vi "Configure Multitone.vi"(0 "VISA resource name":refnum<visa-resource-name>, 1 "Multitone Signal Length (0: ml512)":i32(ring) items=["ml512", "ml1k", "ml2k", "ml4k", "ml8k", "ml16k", "ml32k"], 2 "Number Of Tones (1)":i32=1, 5 "Generator (0: Analog)":i32(ring) items=["Analog", "Digital"], 7 "Output Mode (0: Mono)":i32(ring) items=["Mono", "Stereo"], 9 "Sample Rate (0: mtHz512k)":i32(ring) items=["mtHz512k", "mtHz128k", "mtHz64k", "mtISR", "mtOSR"], 11 "error in (no error)":errorcluster, 12 "Repeat Count (1)":i32=1) -> (4 "VISA resource name out":refnum<visa-resource-name>, 15 "error out":errorcluster)   [LabVIEW 2014, in "Stanford Research SR1.lvlib"]
doc: "Configures the basic attributes for the Multitone."
uses:
  Stanford Research SR1.lvlib
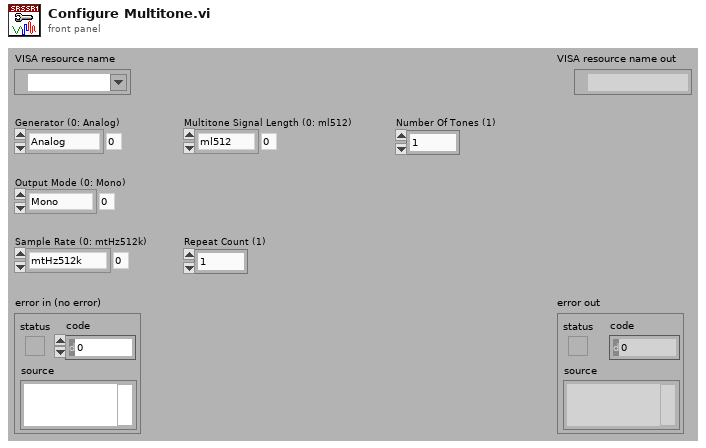
[diagram p1: front panel]
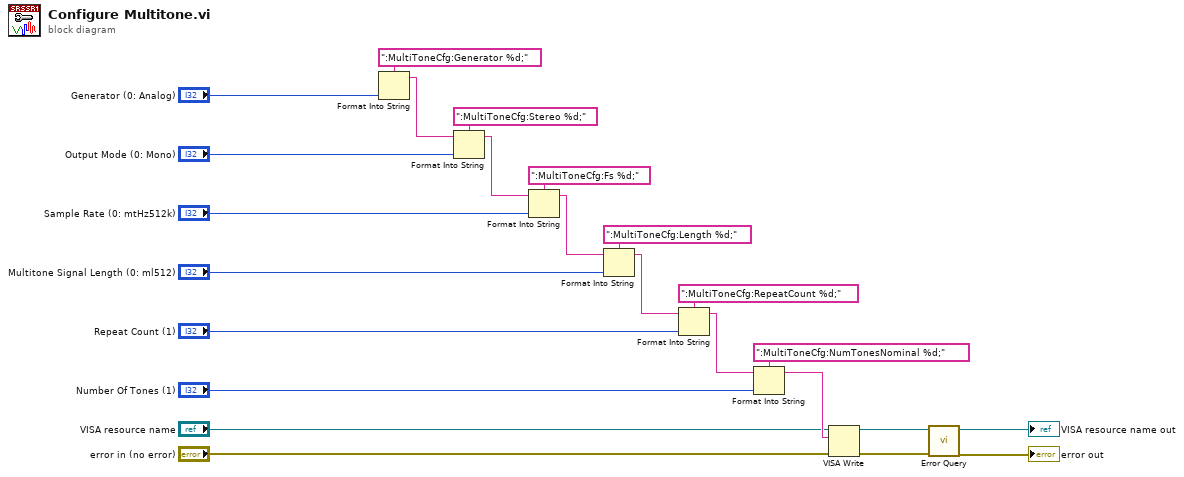
[diagram p0: block diagram]
diagram:
  n1 = Format Into String(format string=":MultiToneCfg:Generator %d;", "Generator (0: Analog)") -> (resulting string=w22:string)  [unwired: 2 in, 1 out]
  n2 = Format Into String(format string=":MultiToneCfg:Stereo %d;", initial string=w22, "Output Mode (0: Mono)") -> (resulting string=w19:string)  [unwired: 1 in, 1 out]
  n3 = Format Into String(format string=":MultiToneCfg:Fs %d;", initial string=w19, "Sample Rate (0: mtHz512k)") -> (resulting string=w16:string)  [unwired: 1 in, 1 out]
  n4 = Format Into String(format string=":MultiToneCfg:Length %d;", initial string=w16, "Multitone Signal Length (0: ml512)") -> (resulting string=w13:string)  [unwired: 1 in, 1 out]
  n5 = Format Into String(format string=":MultiToneCfg:RepeatCount %d;", initial string=w13, "Repeat Count (1)") -> (resulting string=w10:string)  [unwired: 1 in, 1 out]
  n6 = Format Into String(format string=":MultiToneCfg:NumTonesNominal %d;", initial string=w10, "Number Of Tones (1)") -> (resulting string=w7:string)  [unwired: 1 in, 1 out]
  n7 = VISA Write(VISA resource name="VISA resource name", write buffer=w7, error in (no error)="error in (no error)") -> (VISA resource name out=w4:refnum<visa-resource-name>, error out=w3:errorcluster)  [unwired: 1 out]
  n8 = call "Error Query.vi"("error in (no error)"=w3, "VISA resource name"=w4) -> ("error out"=→"error out":errorcluster, "VISA resource name out"=→"VISA resource name out":refnum<visa-resource-name>)  [unwired: 6 in, 2 out]
